vi "gen rf ramp 3 nuclei.vi"(6 "pts":dbl, 8 "span":dbl, 9 "freq3":dbl, 10 "freq2":dbl, 11 "freq1":dbl) -> (3 "freqarray":string[](array[string]))   [LabVIEW 2009]
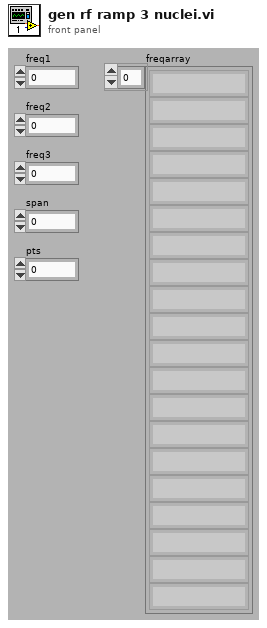
[diagram p1: front panel]
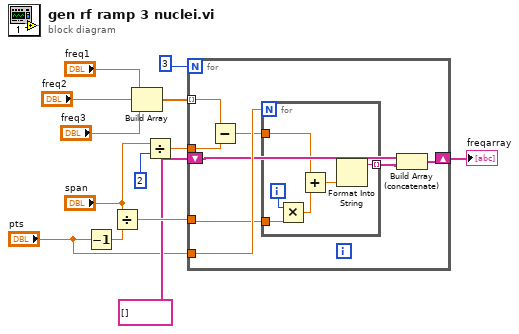
[diagram p0: block diagram]
diagram:
  n1 = Decrement(x="pts") -> (x-1=w2:dbl)
  n2 = Divide(x="span", y=w2) -> (x/y=w5:dbl)
  n3 = Build Array("freq1", "freq2", "freq3") -> (w9:dbl[])
  n4 = Divide(x="span", y=2) -> (x/y=w6:dbl)
  n5 = for {
    N: 3 -> [_]
    tunnel: w9 -> [w21] mode=indexing
    tunnel: w6 -> [w20]
    tunnel: w5 -> [w14]
    tunnel: "pts" -> [w19]
    shift-right: [w17] -> w4
    shift-left: string[] [] -> [w15]
    n6 = Subtract(x=w21, y=w20) -> (x-y=w18:dbl)
    n7 = for {
      N: w19 -> [_]
      tunnel: [w26] -> w16 mode=indexing
      tunnel: w18 -> [w27]
      tunnel: w14 -> [w22]
      i -> [w23]
      n8 = Multiply(x=w23, y=w22) -> (x*y=w24:dbl)
      n9 = Add(x=w27, y=w24) -> (x+y=w25:dbl)
      n10 = Format Into String(w25) -> (resulting string=w26:string)  [unwired: 3 in, 1 out]
    }
    n11 = Build Array (concatenate)(w15, w16) -> (w17:string[])
  }
  "freqarray" <- w4
